vi "Global Torsiometro and SG.vi"() -> ()   [LabVIEW 2019]
panel:
  out "Torsiometro/StrianGauge":bool
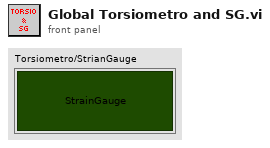
[diagram p1: front panel]
diagram:
